vi "MakeImageTypes.vi"(2 "String In":string, 3 "Action":enum16{"Make string", "Decode string"}(ring)) -> (0 "String Out":string=" ", 1 "ImageTypes":string[](array[string]))   [LabVIEW 2014]
uses:
  globals/AzCamGlobals.vi
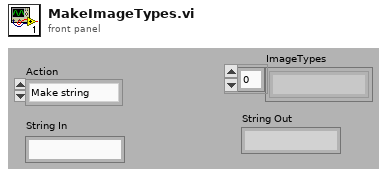
[diagram p1: front panel]
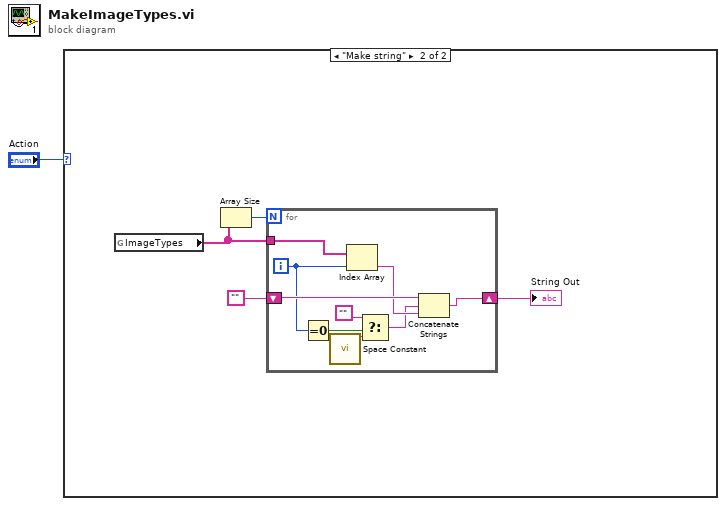
[diagram p0: block diagram]
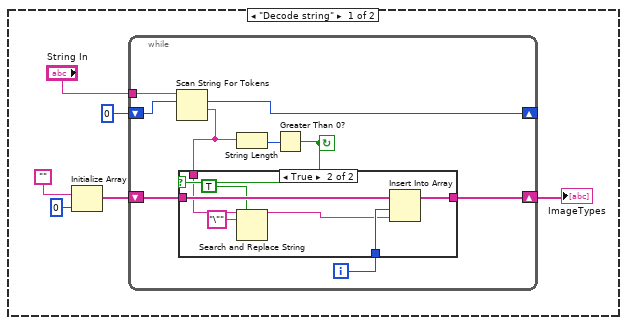
[diagram p2: hidden frame]
diagram:
  n1 = case shown="\"Make string\"" "Action" {
    frame "Decode string" {
      n2 = Initialize Array("", 0 ("dimension size")) -> (w2:string[])
      n3 = while {
        shift-right: [w15] -> _
        shift-left: 0 ("offset") -> [w16]
        shift-right: [w13] -> w5
        shift-left: w2 -> [w14]
        tunnel: "String In" -> [w9]
        i -> [w12]
        stop <- w8 continue-if-true
        n4 = Scan String For Tokens(8:w16, 9:w9) -> (1:w10:string, 2:w15:i32)  [unwired: 4 in, 2 out]
        n5 = String Length(string=w10) -> (length=w11:i32)
        n6 = Greater Than 0?(x=w11) -> (x > 0?=w8:bool)
        n7 = case shown="True" w8 {
          tunnel: w14 -> [w17 w24]
          tunnel: [w17 w23] -> w13
          tunnel: w12 -> [_ w22]
          tunnel: w10 -> [_ w21]
          frame False {
          }
          frame True {
            n8 = Search and Replace String(replace all?=TRUE ("replace all? (F)"), input string=w21, search string="\"") -> (result string=w20:string)  [unwired: 5 in, 3 out]
            n9 = Insert Into Array(array=w24, index=w22, new element=w20) -> (w23:string[])
          }
        }
      }
      "ImageTypes" <- w5
    }
    frame "Make string" {
      n10 = global read "AzCamGlobals.vi" "ImageTypes"() -> (w28:string[])
      n11 = Array Size(array=w28) -> (size(s)=w27:i32)
      n12 = for {
        N: w27 -> [_]
        tunnel: w28 -> [w37]
        shift-right: [w36] -> w25
        shift-left: "" -> [w35]
        i -> [w33]
        n13 = Equal To 0?(x=w33) -> (x = 0?=w32:bool)
        n14 = call <vilib>:"Space Constant.vi"() -> ("String"=w31:string)
        n15 = Index Array(array=w37, index=w33) -> (element=w34:string)
        n16 = Select(t="", s=w32, f=w31) -> (s? t:f=w29:string)
        n17 = Concatenate Strings(w35, w29, w34) -> (w36:string)
      }
      "String Out" <- w25
    }
  }
